vi "Auto_Routine_DepositConeBalance.vi"(8 "error in (no error)":errorcluster, 11 "IsBlue?":bool) -> (0 "error out":errorcluster)   [LabVIEW 2020]
doc: "deposits cone, drives backwards, balances. Starts from 3rd node from non pickup edge. Determines is it is blue or red (by IsBlue?) then changes actions accordingly.\n\ninputs: \n--IsBlue?--Boolean--\n--ErrorIn--\noutputs:\n--ErrorOut--"
uses:
  Arm/ArmGamePiecePreset.ctl
  Arm/ArmPositionPreset.ctl
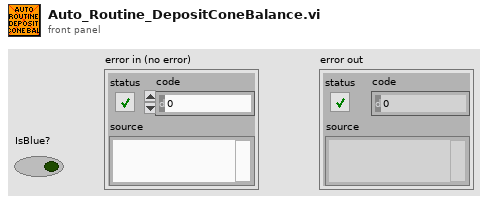
[diagram p1: front panel]
types:
  T1 = typedef "ArmGamePiecePreset.ctl" = enum16{"Cube", "Cone"}
  T2 = typedef "ArmPositionPreset.ctl" = enum16{"Upper", "Lower", "Middle", "Home", "Shelf", "Floor", "HalfFloor", "HalfHome"}
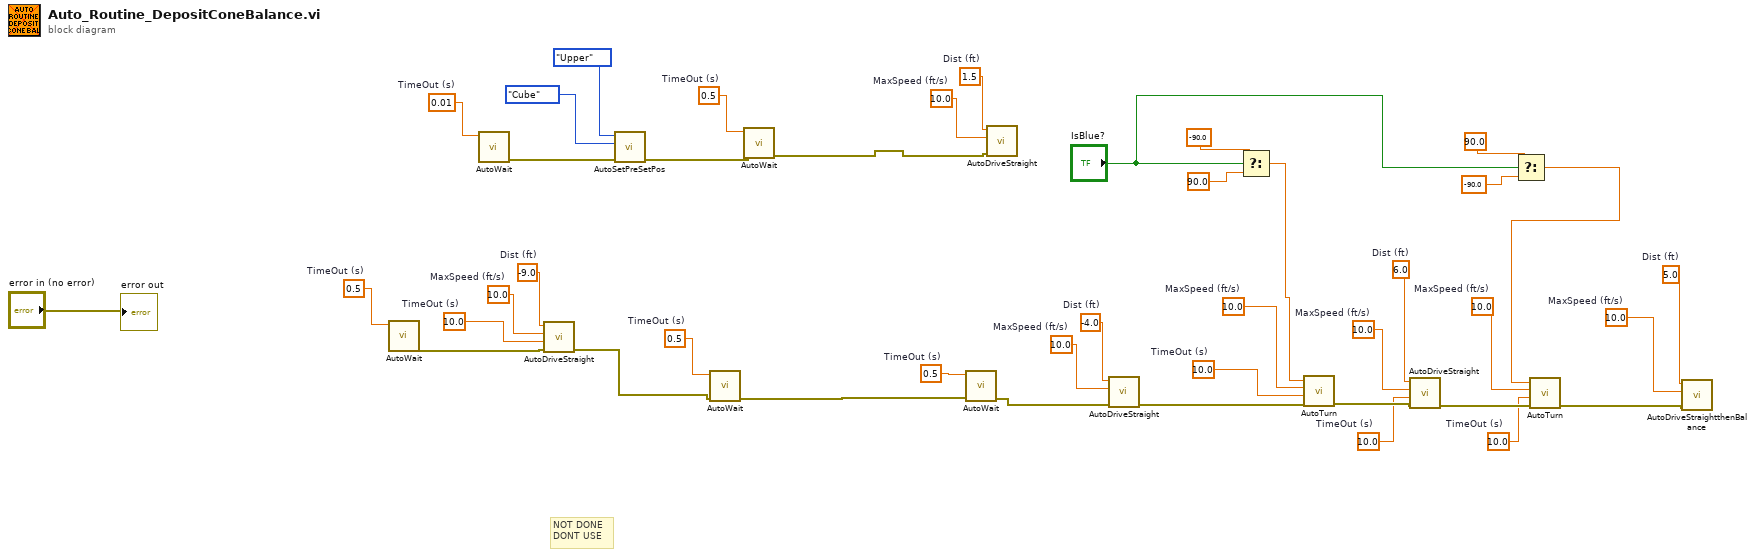
[diagram p0: block diagram]
diagram:
  w2 = 10.0  # TimeOut (s)
  w3 = 10.0  # TimeOut (s)
  w4 = 10.0  # TimeOut (s)
  w5 = 10.0  # TimeOut (s)
  w18 = 10.0  # MaxSpeed (ft/s)
  w19 = 5.0  # Dist (ft)
  w22 = 10.0  # MaxSpeed (ft/s)
  w23 = 10.0  # MaxSpeed (ft/s)
  w24 = 6.0  # Dist (ft)
  w26 = 10.0  # MaxSpeed (ft/s)
  w28 = -4.0  # Dist (ft)
  w29 = 10.0  # MaxSpeed (ft/s)
  w30 = 0.5  # TimeOut (s)
  w31 = 0.5  # TimeOut (s)
  w33 = -9.0  # Dist (ft)
  w34 = 10.0  # MaxSpeed (ft/s)
  w35 = 0.5  # TimeOut (s)
  w36 = 1.5  # Dist (ft)
  w37 = 10.0  # MaxSpeed (ft/s)
  w39 = 0.5  # TimeOut (s)
  w41 = 0.01  # TimeOut (s)
  # "NOT DONE\nDONT USE"
  n1 = call "AutoWait.vi"("TimeOut (s)"=w35) -> ("error out"=w32:errorcluster)  [unwired: 10 in]
  n2 = call "AutoWait.vi"("TimeOut (s)"=w41) -> ("error out"=w40:errorcluster)  [unwired: 10 in]
  n3 = call "AutoDriveStraight.vi"("error in (no error)"=w32, "TimeOut (s)"=w5, "MaxSpeed (ft/s)"=w34, "Dist (ft)"=w33) -> ("error out"=w15:errorcluster)  [unwired: 7 in]
  n4 = call "AutoSetPreSetPos.vi"("error in (no error)"=w40, "Game Piece"=ArmGamePiecePreset."Cube", "Position"=ArmPositionPreset."Upper") -> ("error out"=w38:errorcluster)  [unwired: 6 in, 2 out]
  n5 = call "AutoWait.vi"("error in (no error)"=w15, "TimeOut (s)"=w31) -> ("error out"=w1:errorcluster)  [unwired: 9 in]
  n6 = call "AutoWait.vi"("error in (no error)"=w38, "TimeOut (s)"=w39) -> ("error out"=w14:errorcluster)  [unwired: 9 in]
  n7 = call "AutoWait.vi"("error in (no error)"=w1, "TimeOut (s)"=w30) -> ("error out"=w13:errorcluster)  [unwired: 9 in]
  n8 = call "AutoDriveStraight.vi"("error in (no error)"=w14, "MaxSpeed (ft/s)"=w37, "Dist (ft)"=w36) -> ()  [unwired: 8 in, 1 out]
  n9 = call "AutoDriveStraight.vi"("error in (no error)"=w13, "MaxSpeed (ft/s)"=w29, "Dist (ft)"=w28) -> ("error out"=w27:errorcluster)  [unwired: 8 in]
  n10 = Select(t=-90.0, s="IsBlue?", f=90.0) -> (s? t:f=w7:dbl)
  n11 = call "AutoTurn.vi"("error in (no error)"=w27, "TimeOut (s)"=w4, "MaxSpeed (ft/s)"=w26, "degrees"=w7) -> ("error out"=w25:errorcluster)  [unwired: 7 in]
  n12 = call "AutoDriveStraight.vi"("error in (no error)"=w25, "TimeOut (s)"=w3, "MaxSpeed (ft/s)"=w23, "Dist (ft)"=w24) -> ("error out"=w21:errorcluster)  [unwired: 7 in]
  n13 = Select(t=90.0, s="IsBlue?", f=-90.0) -> (s? t:f=w8:dbl)
  n14 = call "AutoTurn.vi"("error in (no error)"=w21, "TimeOut (s)"=w2, "MaxSpeed (ft/s)"=w22, "degrees"=w8) -> ("error out"=w20:errorcluster)  [unwired: 7 in]
  n15 = call "AutoDriveStraightthenBalance.vi"("error in (no error)"=w20, "MaxSpeed (ft/s)"=w18, "Dist (ft)"=w19) -> ()  [unwired: 8 in, 1 out]
  "error out" <- "error in (no error)"
